vi "ApplyColorTransformation.vi"(9 "Cluster in":cluster{i32, i32, i32}, 10 "Image Pixels (U32)":u32[][](array[numeric]), 11 "Refnum in":T1) -> (3 "Refnum out":T1)   [LabVIEW 2019]
uses:
  <vilib>/vision/Image Controls.llb/IMAQ Image.ctl
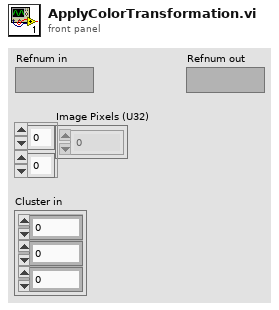
[diagram p1: front panel]
types:
  T1 = typedef "IMAQ Image.ctl" = refnum<image>
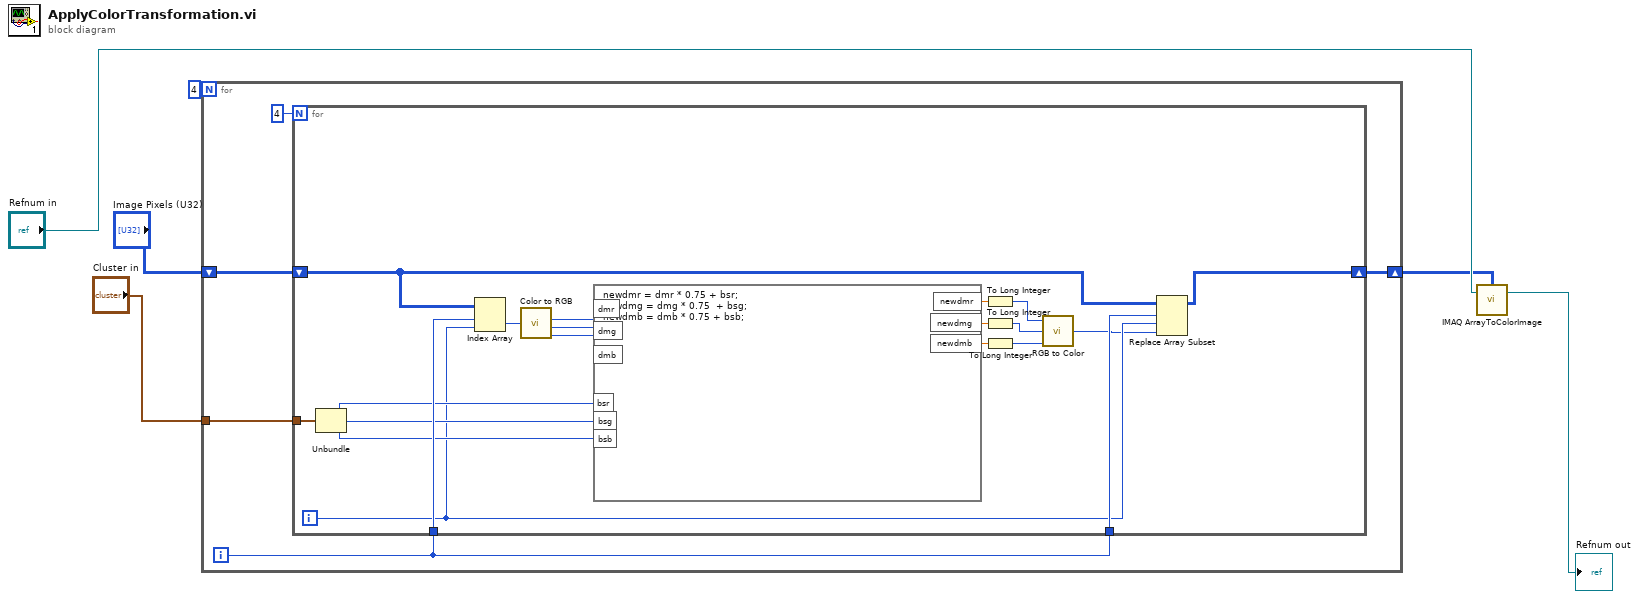
[diagram p0: block diagram]
diagram:
  n1 = for {
    N: 4 -> [_]
    tunnel: "Cluster in" -> [w10]
    shift-right: [w8] -> w4
    shift-left: "Image Pixels (U32)" -> [w9]
    i -> [w7]
    n2 = for {
      N: 4 -> [_]
      tunnel: w7 -> [w31]
      tunnel: w10 -> [w23]
      shift-right: [w18] -> w8
      shift-left: w9 -> [w22]
      tunnel: w7 -> [w21]
      i -> [w20]
      n3 = Unbundle(w23) -> (w30:i32, w29:i32, w28:i32)
      n4 = Index Array(array=w22, index (row)=w31, index (col)=w20) -> (element=w27:u32)
      n5 = call <vilib>:"Color to RGB.vi"("Color"=w27) -> ("R"=w26:u8, "G"=w25:u8, "B"=w24:u8)  [unwired: 1 out]
      n6 = formula code="newdmr = dmr * 0.75 + bsr;\nnewdmg = dmg * 0.75  + bsg;\nnewdmb = dmb * 0.75 + bsb;"("bsr"=w30, "bsg"=w29, "bsb"=w28, "dmr"=w26, "dmg"=w25, "dmb"=w24) -> ("newdmr"=w17:dbl, "newdmg"=w16:dbl, "newdmb"=w15:dbl)
      n7 = To Long Integer(number=w17) -> (32bit integer=w12:i32)
      n8 = To Long Integer(number=w16) -> (32bit integer=w13:i32)
      n9 = To Long Integer(number=w15) -> (32bit integer=w14:i32)
      n10 = call <vilib>:"RGB to Color.vi"("B"=w14, "G"=w13, "R"=w12) -> ("Color"=w19:u32)
      n11 = Replace Array Subset(array=w22, new element=w19, index (row)=w21, index (col)=w20) -> (w18:u32[][])
    }
  }
  n12 = call "IMAQ ArrayToColorImage"("Image Pixels (U32)"=w4, "Image"="Refnum in") -> ("Image Out"=→"Refnum out":T1)  [unwired: 3 in, 1 out]
